vi "LabVIEWWebsocketMessages - Single Connection.vi"() -> ()   [LabVIEW 2014]
uses:
  <vilib>/Intelligent Energy/WebSockets API/WebSockets/WebSockets.lvlib
panel:
  out "LED 2":bool
  out "LED 1":bool
  out "User Text (Log)":string="\r\n"
  out "User Text (Last)":string
  out "data (default)":string
  out "msg (default)":string="ssssss"
  out "data (JSON) 2":string
  out "msg (string)":string="Core : CN Close"
  in  "Toggle LED 2":bool
  in  "Toggle LED 1":bool
  out "Request URI":string="/"
  out "HTTP Headers":variant=variant("Accept"=variant(string "text/html,application/xhtml+xml,application/xml;q=0.9,*/*;q=0.8"), "Accept-Encoding"=variant(string "gzip, deflate"), "Accept-Language"=variant(string "en-GB,en;q=0.5"), "Cache-Control"=variant(string "no-cache"), "Connection"=variant(string "keep-alive, Upgrade"), "DNT"=variant(string "1"), "Host"=variant(string "localhost:6125"), "Origin"=variant(string "http://localhost:8000"), "Pragma"=variant(string "no-cache"), "Sec-WebSocket-Extensions"=variant(string "permessage-deflate"), "Sec-WebSocket-Key"=variant(string "dPMfcRTFpHjstnxySTdG7A=="), "Sec-WebSocket-Version"=variant(string "13"), "Upgrade"=variant(string "websocket"), "User-Agent"=variant(string "Mozilla/5.0 (Windows NT 10.0; WOW64; rv:42.0) Gecko/20100101 Firefox/42.0"))
  in  "Stop":bool
  in  "Send":bool
  in  "Message":string="new message"
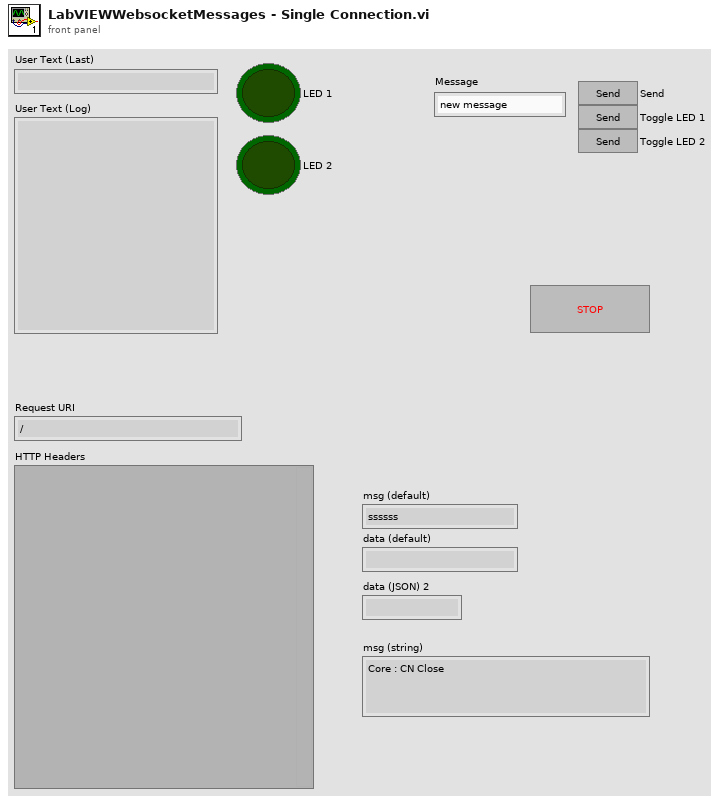
[diagram p1: front panel]
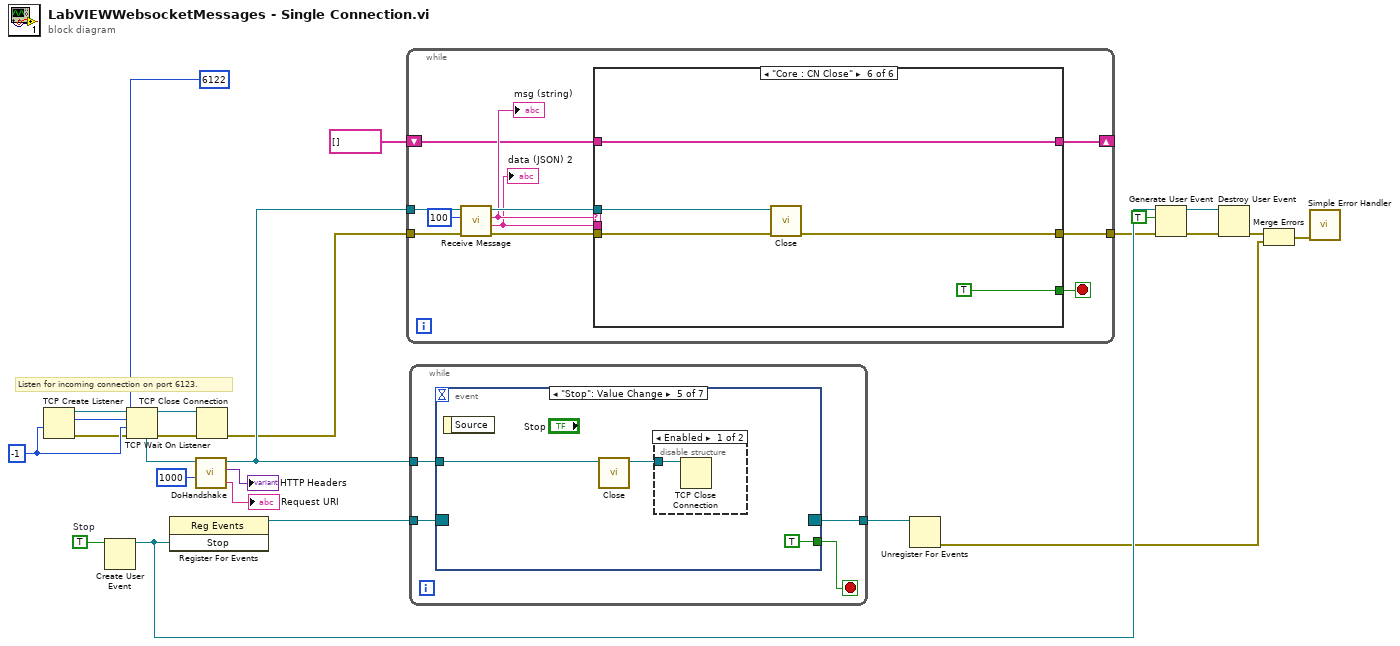
[diagram p0: block diagram]
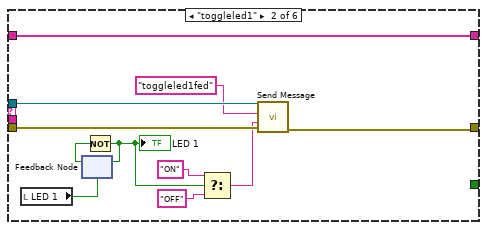
[diagram p3: hidden frame]
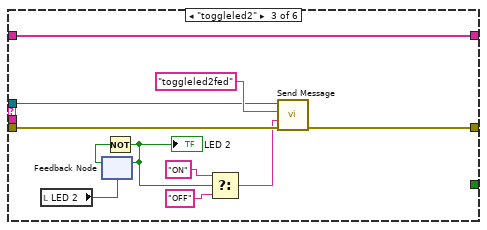
[diagram p4: hidden frame]
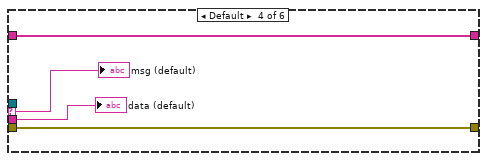
[diagram p5: hidden frame]
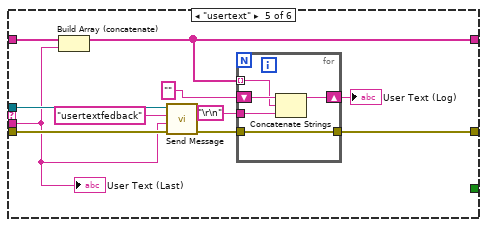
[diagram p6: hidden frame]
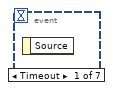
[diagram p7: hidden frame]
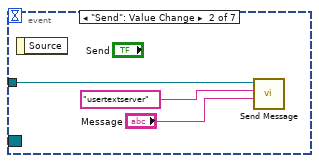
[diagram p8: hidden frame]
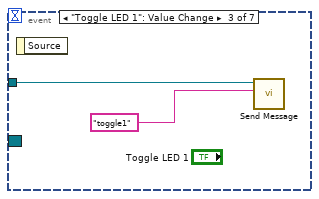
[diagram p9: hidden frame]
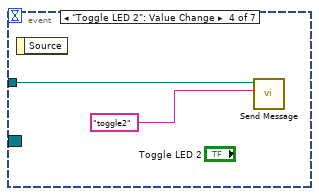
[diagram p10: hidden frame]
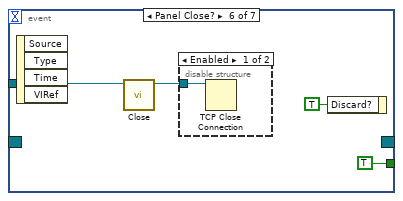
[diagram p12: hidden frame]
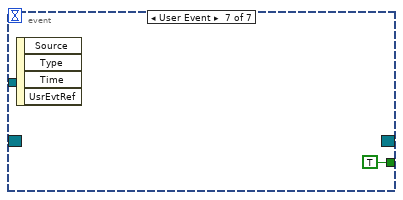
[diagram p14: hidden frame]
diagram:
  w15 = TRUE  # Stop
  w22 = -1 ("timeout ms (25000)")
  # "Listen for incoming connection on port 6123."
  n1 = TCP Create Listener(9:w22, 10:u16 6122 ("port")) -> (0:w20:errorcluster, 3:w21:refnum<k5>)  [unwired: 3 in, 1 out]
  n2 = Create User Event(user event datatype=w15) -> (user event=w13:refnum<user-event>)  [unwired: 1 in, 1 out]
  n3 = TCP Wait On Listener(8:w20, 9:w22, 11:w21) -> (0:w17:errorcluster, 3:w18:refnum<k5>, 4:w19:refnum<k5>)  [unwired: 1 in, 2 out]
  n4 = register-events(w13) -> (reference out=w16:refnum<event-registration>)  [unwired: 2 in, 1 out]
  n5 = call <vilib>:"DoHandshake.vi"("timeout ms (5000)"=1000 ("timeout ms (25000)"), "WebSocket Connection in"=w19) -> ("Request URI"=→"Request URI":string, "Headers Out"=→"HTTP Headers":variant, "WebSocket Connection out"=w24:refnum<k5>)  [unwired: 6 in, 1 out]
  n6 = TCP Close Connection(connection ID=w18, error in (no error)=w17) -> (error out=w4:errorcluster)  [unwired: 1 in, 1 out]
  n7 = while {
    tunnel: w24 -> [w35]
    tunnel: w4 -> [w34]
    tunnel: [w28] -> w3
    shift-right: [w26] -> _
    shift-left: string[] [] ("appended array") -> [w25]
    stop <- w27 stop-if-true
    n8 = call "Receive Message.vi"("error in (no error)"=w34, "timeout ms (5000)"=100, "WebSocket Connection in"=w35) -> ("error out"=w32:errorcluster, "data (JSON)"=w29:string, "msg (string)"=w30:string, "WebSocket Connection out"=w31:refnum<k5>)  [unwired: 5 in]
    "msg (string)" <- w30
    "data (JSON) 2" <- w29
    n9 = case shown="\"Core : CN Close\"" w30 {
      selector: w30 -> [_ _ _ w62 _ _]
      tunnel: w32 -> [w37 w45 w55 w63 w69 w83]
      tunnel: w31 -> [_ w43 w54 _ w67 w81]
      tunnel: w29 -> [_ _ _ w61 w65 _]
      tunnel: [w37 w44 w53 w63 w71 w82] -> w28
      tunnel: [_ _ _ _ _ TRUE] -> w27
      tunnel: [w36 w48 w59 w60 w73 w80] -> w26
      tunnel: w25 -> [w36 w48 w59 w60 w74 w80]
      frame "Core :Timeout" {
      }
      frame "toggleled1" {
        n10 = local read "LED 1"() -> (w47:bool)
        n11 = feedback #1(w47) -> (w46:bool)
        n12 = Not(x=w46) -> (.not. x?=w40:bool)
        "LED 1" <- w40
        n13 = feedback-in #1(w40) -> ()
        n14 = Select(t="ON", s=w40, f="OFF") -> (s? t:f=w38:string)
        n15 = call "Send Message.vi"("error in (no error)"=w45, "data (JSON)"=w38, "msg (string)"="toggleled1fed", "WebSocket Connection in"=w43) -> ("error out"=w44:errorcluster)  [unwired: 6 in, 1 out]
      }
      frame "toggleled2" {
        n16 = local read "LED 2"() -> (w58:bool)
        n17 = feedback #2(w58) -> (w57:bool)
        n18 = Not(x=w57) -> (.not. x?=w50:bool)
        "LED 2" <- w50
        n19 = feedback-in #2(w50) -> ()
        n20 = Select(t="ON", s=w50, f="OFF") -> (s? t:f=w49:string)
        n21 = call "Send Message.vi"("error in (no error)"=w55, "data (JSON)"=w49, "msg (string)"="toggleled2fed", "WebSocket Connection in"=w54) -> ("error out"=w53:errorcluster)  [unwired: 6 in, 1 out]
      }
      frame Default {
        "msg (default)" <- w62
        "data (default)" <- w61
      }
      frame "usertext" {
        n22 = Build Array (concatenate)(w74, w65) -> (w73:string[])
        n23 = call "Send Message.vi"("error in (no error)"=w69, "data (JSON)"=w65, "msg (string)"="usertextfedback", "WebSocket Connection in"=w67) -> ("error out"=w68:errorcluster)  [unwired: 6 in, 1 out]
        n24 = for {
          tunnel: w73 -> [w77] mode=indexing
          shift-right: [w79] -> w70
          shift-left: "" -> [w78]
          tunnel: "\r\n" -> [w76]
          tunnel: w68 -> [w75]
          tunnel: [w75] -> w71
          n25 = Concatenate Strings(w78, w77, w76) -> (w79:string)
        }
        "User Text (Log)" <- w70
        "User Text (Last)" <- w65
      }
      frame "Core : CN Close" {
        n26 = call <vilib>:"Close.vi"("error in (no error)"=w83, "WebSocket Connection in"=w81) -> ("error out"=w82:errorcluster)  [unwired: 8 in, 1 out]
      }
    }
  }
  n27 = while {
    tunnel: w24 -> [w88]
    tunnel: w16 -> [w86]
    tunnel: [w85] -> w14
    stop <- w87 stop-if-true
    n28 = event shown="[4] \"Stop\": Value Change" {
      selector: w86 -> [_ _ _ _ _ _ _]
      dyn-events: [_ _ _ _ _ _ _] -> w85
      timeout: _ -> [_ _ _ _ _ _ _]
      tunnel: w88 -> [_ w91 w93 w95 w97 w102 _]
      tunnel: [_ _ _ _ TRUE TRUE TRUE] -> w87
      event Timeout {
        n29 = event-data() -> ()  [unwired: 1 in, 1 out]
      }
      event "Send": Value Change {
        n30 = event-data() -> ()  [unwired: 1 in, 1 out]
        n31 = call "Send Message.vi"("data (JSON)"="Message", "msg (string)"="usertextserver", "WebSocket Connection in"=w91) -> ()  [unwired: 7 in, 2 out]
      }
      event "Toggle LED 1": Value Change {
        n32 = event-data() -> ()  [unwired: 1 in, 1 out]
        n33 = call "Send Message.vi"("msg (string)"="toggle1" ("Message 2"), "WebSocket Connection in"=w93) -> ()  [unwired: 8 in, 2 out]
      }
      event "Toggle LED 2": Value Change {
        n34 = event-data() -> ()  [unwired: 1 in, 1 out]
        n35 = call "Send Message.vi"("msg (string)"="toggle2" ("Message 2"), "WebSocket Connection in"=w95) -> ()  [unwired: 8 in, 2 out]
      }
      event "Stop": Value Change {
        n36 = event-data() -> ()  [unwired: 1 in, 1 out]
        n37 = call <vilib>:"Close.vi"("WebSocket Connection in"=w97) -> ("WebSocket Connection in"=w96:refnum<k5>)  [unwired: 9 in, 1 out]
        n38 = disable-structure shown="Enabled" {
          disable-tunnel: w96 -> [w99 _]
          frame Enabled {
            n39 = TCP Close Connection(connection ID=w99) -> ()  [unwired: 2 in, 2 out]
          }
          frame Disabled {
          }
        }
      }
      event Panel Close? {
        n40 = event-data() -> ()  [unwired: 1 in, 4 out]
        n41 = call <vilib>:"Close.vi"("WebSocket Connection in"=w102) -> ("WebSocket Connection in"=w101:refnum<k5>)  [unwired: 9 in, 1 out]
        n42 = disable-structure shown="Enabled" {
          disable-tunnel: w101 -> [w104 _]
          frame Enabled {
            n43 = TCP Close Connection(connection ID=w104) -> ()  [unwired: 2 in, 2 out]
          }
          frame Disabled {
          }
        }
        n44 = event-data("Discard?"=TRUE) -> ()  [unwired: 1 in, 1 out]
      }
      event User Event {
        n45 = event-data() -> ()  [unwired: 1 in, 4 out]
      }
    }
  }
  n46 = Unregister For Events(event registration refnum=w14) -> (error out=w9:errorcluster)  [unwired: 1 in]
  n47 = Generate User Event(user event=w13, event data cluster=TRUE ("event data"), error in=w3) -> (user event out=w12:refnum<user-event>, error out=w11:errorcluster)  [unwired: 1 in]
  n48 = Destroy User Event(user event=w12, error in=w11) -> (error out=w10:errorcluster)
  n49 = Merge Errors(w10, w9) -> (w5:errorcluster)
  n50 = call <vilib>:"Simple Error Handler.vi"("error in (no error)"=w5) -> ()  [unwired: 4 in, 5 out]
